vi "PrjPath_Read.vi"(7 "error in (no error)":errorcluster caption="错误输入（无错误）") -> (0 "error out":errorcluster caption="错误输出", 1 "Valid":bool, 2 "Path":path)   [LabVIEW 2016]
uses:
  <vilib>/Utility/config.llb/Read Key (Path).vi
  <vilib>/Utility/config.llb/NI_LVConfig.lvlib
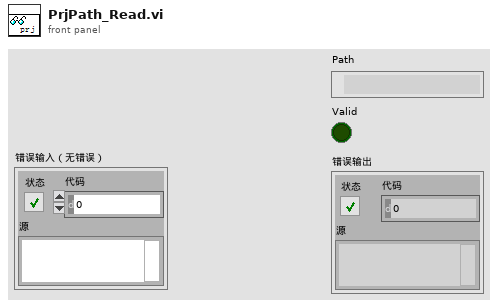
[diagram p1: front panel]
types:
  T1 = cluster{"TREE PNG":path, "User Guide":path, "DefaultSave":path, "BuildPath":path, "Image":path, "Modules":path, "Configuration":path, "License":path, "SplitFiles":path, "System.ini":path}
  T2 = typedef "NI_LVConfig.lvlib/Config Data RefNum.ctl" = refnum<k1>
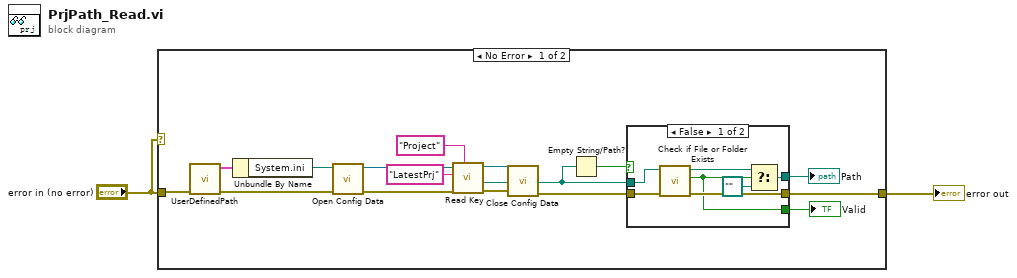
[diagram p0: block diagram]
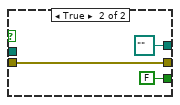
[diagram p2: hidden frame]
diagram:
  n1 = case shown="No Error" "error in (no error)" {
    tunnel: [w7 w28] -> w2
    tunnel: "error in (no error)" -> [w9 w28]
    frame No Error {
      n2 = call "UserDefinedPath.vi"() -> ("UserDefinedPath"=w17:T1)  [unwired: 11 in]
      n3 = Unbundle By Name(w17) -> ("System.ini"=w16:path)
      n4 = call <vilib>:"Open Config Data.vi"("error in (no error)"=w9, "configuration file path"=w16) -> ("error out"=w14:errorcluster, "refnum"=w15:T2)  [unwired: 7 in, 1 out]
      n5 = call-poly <vilib>:"Read Key.vi"("section"="Project", "error in (no error)"=w14, "key"="LatestPrj", "refnum"=w15) -> ("error out"=w12:errorcluster, "value"=w5:path, "refnum out"=w13:T2)  [unwired: 4 in, 1 out]
      n6 = call <vilib>:"Close Config Data.vi"("error in (no error)"=w12, "refnum"=w13) -> ("error out"=w8:errorcluster)  [unwired: 8 in, 1 out]
      n7 = Empty String/Path?(string/path=w5) -> (empty?=w4:bool)
      n8 = case shown="False" w4 {
        tunnel: w8 -> [w24 w26]
        tunnel: [w23 w26] -> w7
        tunnel: [w21 path "" ("f")] -> w6
        tunnel: w5 -> [w19 _]
        tunnel: [w18 FALSE ("file or folder exists?")] -> w3
        frame False {
          n9 = call <vilib>:"Check if File or Folder Exists.vi"("error in (no error)"=w24, "path"=w19) -> ("error out"=w23:errorcluster, "file or folder exists?"=w18:bool, "dup path"=w22:path)  [unwired: 7 in]
          n10 = Select(t=w22, s=w18, f=path "") -> (s? t:f=w21:path)
        }
        frame True {
        }
      }
      "Path" <- w6
      "Valid" <- w3
    }
    frame Error {
    }
  }
  "error out" <- w2
